vi "LiftOpen.vi"(6 "Controller Values":T1, 8 "error in (no error)":errorcluster, 11 "Lift in":refnum<class "Lift.lvclass">) -> (0 "error out":errorcluster, 3 "Lift out":refnum<class "Lift.lvclass">)   [LabVIEW 2018, in "Lift.lvclass"]
uses:
  Lift.lvclass
  Lift.lvclass/Lift.ctl
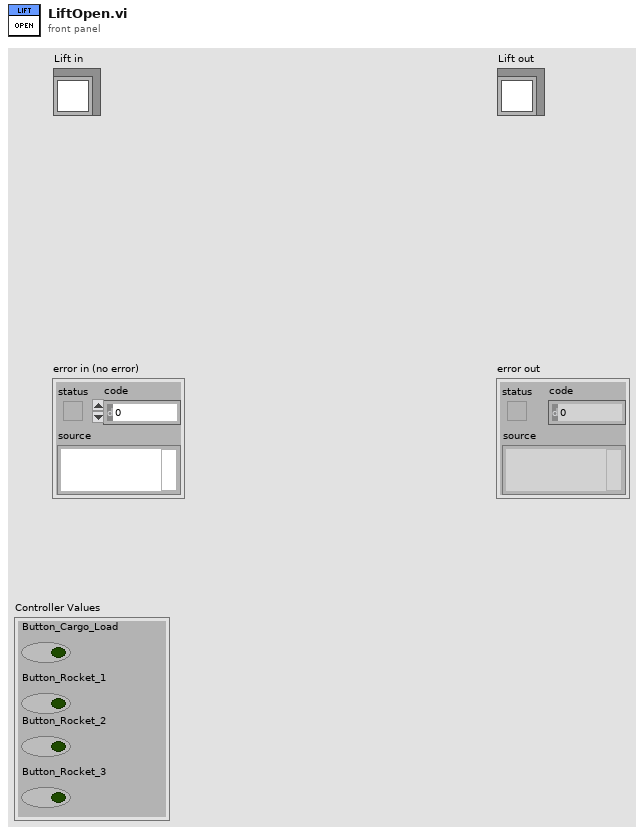
[diagram p1: front panel]
types:
  T1 = cluster{"Button_Cargo_Load":bool, "Button_Rocket_1":bool, "Button_Rocket_2":bool, "Button_Rocket_3":bool}
  T2 = typedef "WPI_MotorControlDeviceRef.ctl" = cluster{"DeviceStatus":errorcluster, "Type":T3, "PWM":cluster{"PWM Channel":T4, "DeadBand":T5}, "CAN":cluster{"Device Number":u8, "SetOutput VI Ref":variant, "GetOutput VI Ref":variant, "Enable VI Ref":variant, "Disable VI Ref":variant, "Data":variant}, "Invert":bool, "DIO PWM":cluster{"PWM \"Enable\" Channel":T4, "DIOChannel":T6, "PWM Rate":dbl}}
  T3 = typedef "WPI_MotorControlType.ctl" = enum16{"PWM", "CAN", "DIO PWM"}
  T4 = typedef "FPGA_DIOPWMChannel.ctl" = enum8{"PWM 0", "PWM 1", "PWM 2", "PWM 3", "PWM 4", "PWM 5", "PWM 6", "PWM 7", "PWM 8", "PWM 9", "PWM MXP 0", "PWM MXP 1", "PWM MXP 2", "PWM MXP 3", "PWM MXP 4", "PWM MXP 5", "PWM MXP 6", "PWM MXP 7", "PWM MXP 8", "PWM MXP 9", "Invalid"}
  T5 = typedef "WPI_PWMDeadband.ctl" = cluster{"Name":string, "maxPositivePwm":i32, "minPositivePwm":i32, "centerPwm":i32, "maxNegativePwm":i32, "minNegativePwm":i32, "angularRange":u16}
  T6 = typedef "FPGA_DIOChannel.ctl" = enum8{"DIO 0", "DIO 1", "DIO 2", "DIO 3", "DIO 4", "DIO 5", "DIO 6", "DIO 7", "DIO 8", "DIO 9", "DIO MXP 0", "DIO MXP 1", "DIO MXP 2", "DIO MXP 3", "DIO MXP 4", "DIO MXP 5", "DIO MXP 6", "DIO MXP 7", "DIO MXP 8", "DIO MXP 9", "DIO MXP 10", "DIO MXP 11", "DIO MXP 12", "DIO MXP 13", "DIO MXP 14", "DIO MXP 15", "SPI Port CS1", "SPI Port CS2", "SPI Port CS3", "SPI Port MISO", "SPI Port MOSI", "Invalid"}
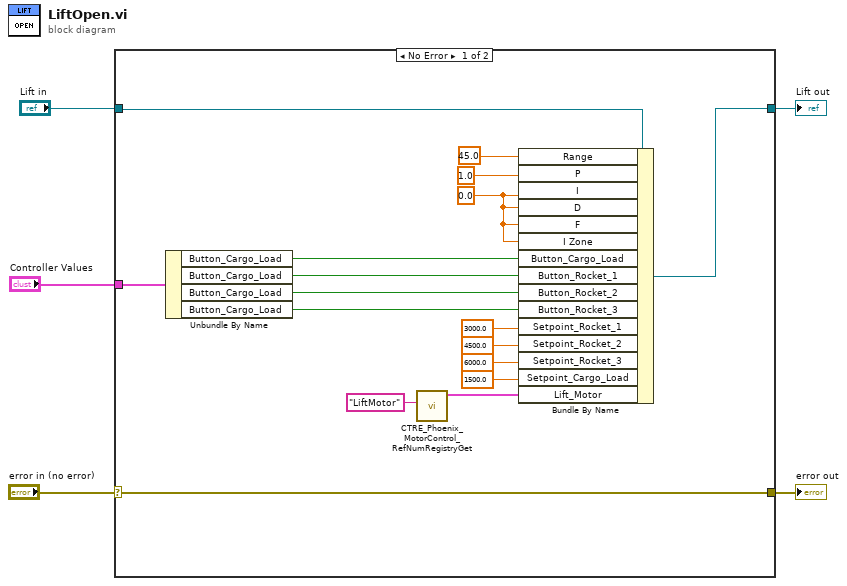
[diagram p0: block diagram]
diagram:
  n1 = case shown="No Error" "error in (no error)" {
    selector: "error in (no error)" -> [w22 w24]
    tunnel: [w22 w24] -> w4
    tunnel: [w6 w23] -> w2
    tunnel: "Lift in" -> [w7 w23]
    tunnel: "Controller Values" -> [w8 _]
    frame No Error {
      w20 = 0.0 ("I")
      n2 = Unbundle By Name(w8) -> ("Button_Cargo_Load"=w12:bool, "Button_Cargo_Load"=w11:bool, "Button_Cargo_Load"=w10:bool, "Button_Cargo_Load"=w9:bool)
      n3 = call <vilib>:"CTRE_Phoenix_MotorControl_RefNumRegistryGet.vi"("refnum name"="LiftMotor") -> ("PhoenixMotorControlDevRef"=w17:T2)  [unwired: 9 in, 1 out]
      n4 = Bundle By Name(cluster=w7, "Range"=45.0 ("P"), "P"=1.0, "I"=w20, "D"=w20, "F"=w20, "I Zone"=w20, "Button_Cargo_Load"=w12, "Button_Rocket_1"=w11, "Button_Rocket_2"=w10, "Button_Rocket_3"=w9, "Setpoint_Rocket_1"=3000.0, "Setpoint_Rocket_2"=4500.0, "Setpoint_Rocket_3"=6000.0, "Setpoint_Cargo_Load"=1500.0, "Lift_Motor"=w17) -> (w6:refnum<class "Lift.lvclass">)
    }
    frame Error {
    }
  }
  "error out" <- w4
  "Lift out" <- w2
